vi "Add Properties to Node.vi"(8 "error in":errorcluster, 10 "Tree Reference":refnum<vi>, 11 "Parent Node":string) -> (0 "error out":errorcluster)   [LabVIEW 2025]
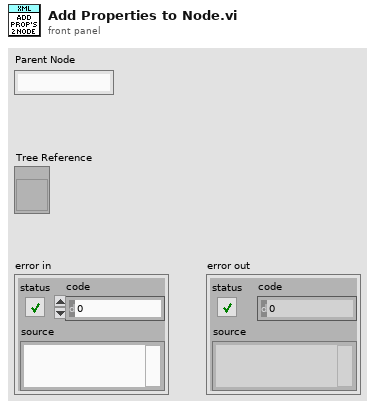
[diagram p1: front panel]
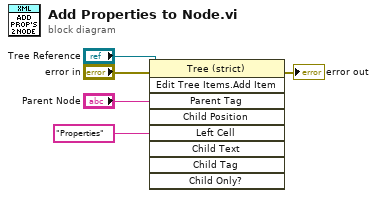
[diagram p0: block diagram]
diagram:
  n1 = invoke on="Invoke Node" class="Tree (strict)" method="Edit Tree Items.Add Item"(reference="Tree Reference", error in="error in", "Parent Tag"="Parent Node", "Left Cell"="Properties" ("Left Cell String")) -> (error out=→"error out":errorcluster)  [unwired: 5 in, 8 out]
